vi "Subvi iterator.vi"(9 "Set increase":bool, 10 "Iterator in":i32, 11 "Nmax":i32) -> (2 "Iterator out":i32)   [LabVIEW 2017]
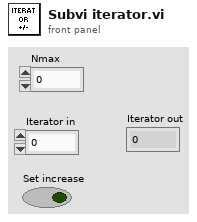
[diagram p1: front panel]
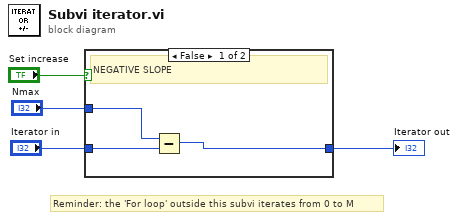
[diagram p0: block diagram]
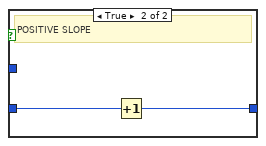
[diagram p2: hidden frame]
diagram:
  # "Reminder: the 'For loop' outside this subvi iterates from 0 to M"
  n1 = case shown="False" "Set increase" {
    tunnel: "Iterator in" -> [w6 w9]
    tunnel: [w5 w8] -> w1
    tunnel: "Nmax" -> [w7 _]
    frame False {
      # "NEGATIVE SLOPE"
      n2 = Subtract(x=w7, y=w6) -> (x-y=w5:i32)
    }
    frame True {
      # "POSITIVE SLOPE"
      n3 = Increment(x=w9) -> (x+1=w8:i32)
    }
  }
  "Iterator out" <- w1
